vi "Untitled 10 (SubVI).vi"(6 "Fuel (kg/s)":dbl, 7 "PID gains":T1={"proportional gain (Kc)"=1.0, "integral time (Ti, min)"=0.01, "derivative time (Td, min)"=0.0} {"derivative time (Td, min)" format="%.3f"; "integral time (Ti, min)" format="%.3f"; "proportional gain (Kc)" format="%.3f"}, 9 "Fuel Control   (On/OFF)":bool, 10 "Numeric":dbl, 11 "Max T (K)":dbl) -> (3 "output":dbl)   [LabVIEW 2019]
uses:
  <vilib>/addons/control/pid/pid.llb/PID Advanced (DBL).vi
  <vilib>/addons/control/pid/NI_PID_pid.lvlib
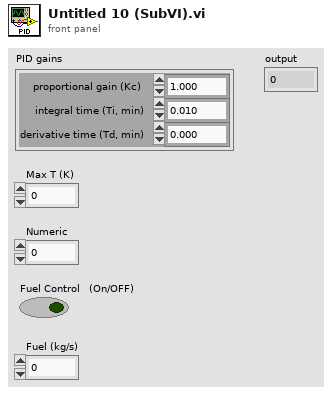
[diagram p1: front panel]
types:
  T1 = cluster{"proportional gain (Kc)":dbl, "integral time (Ti, min)":dbl, "derivative time (Td, min)":dbl}
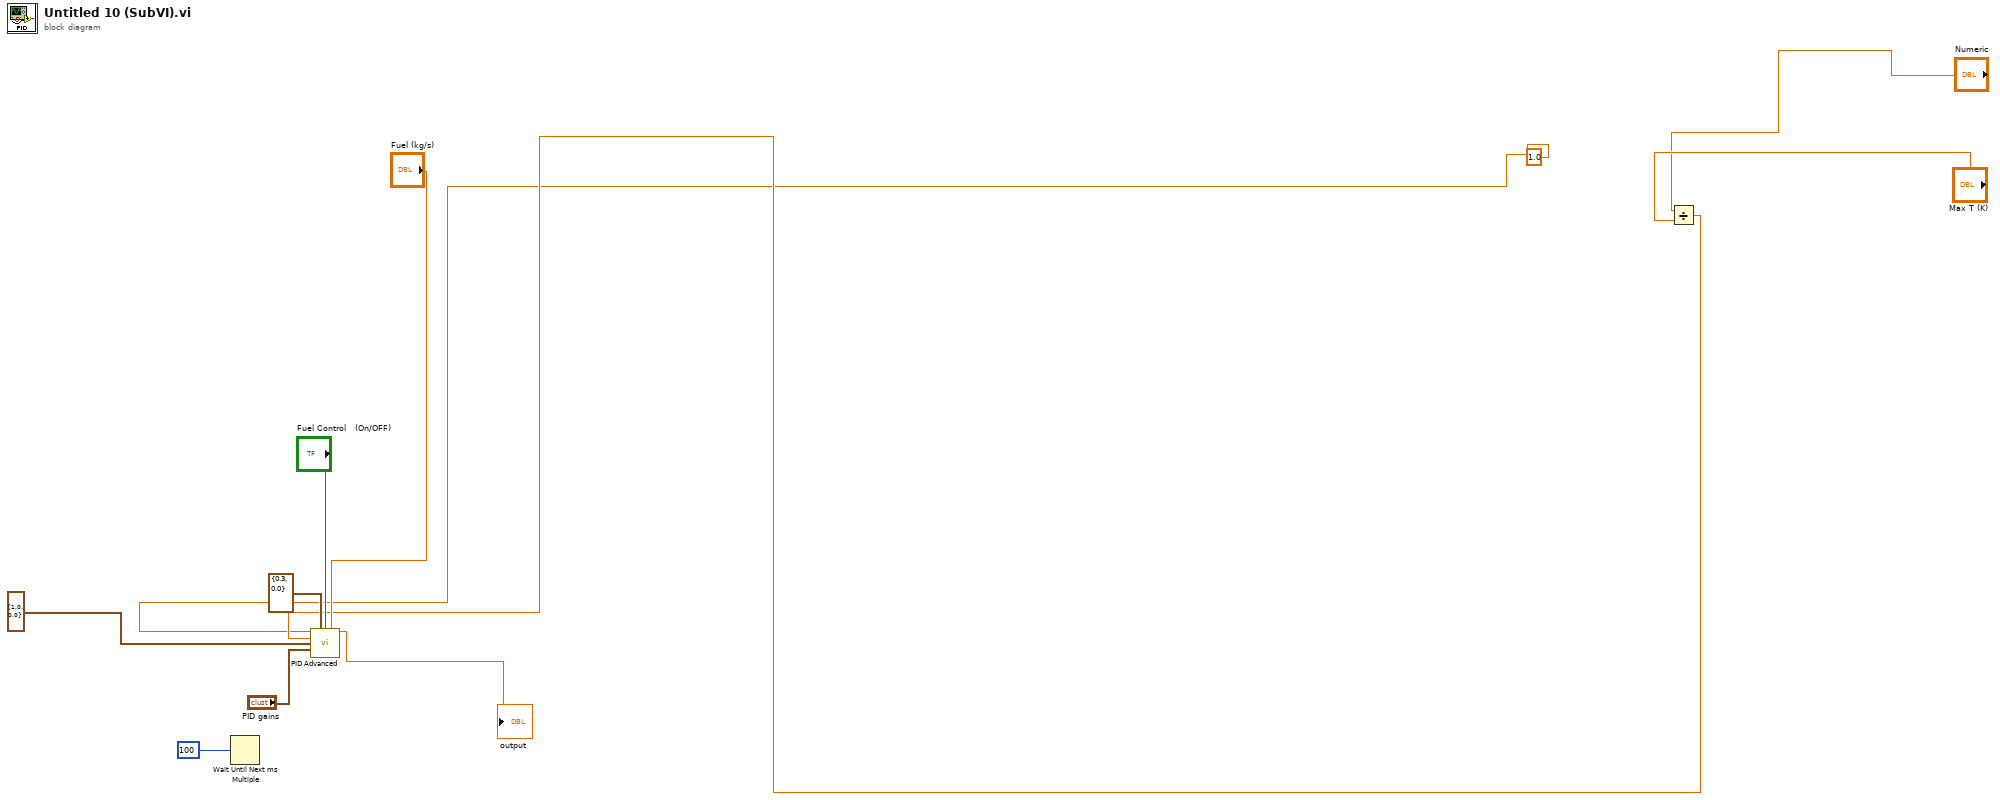
[diagram p0: block diagram]
diagram:
  n1 = Wait Until Next ms Multiple(millisecond multiple=100) -> ()  [unwired: 1 out]
  n2 = Divide(x="Numeric", y="Max T (K)") -> (x/y=w3:dbl)
  n3 = call-poly <vilib>:"PID Advanced.vi"("setpoint"=1.0, "output range"=cluster{"output high":dbl, "output low":dbl} {"output high"=0.3, "output low"=0.0}, "auto? (T)"="Fuel Control   (On/OFF)", "manual control"="Fuel (kg/s)", "process variable"=w3, "setpoint range"=cluster{"setpoint high":dbl, "setpoint low":dbl} {"setpoint high"=1.0, "setpoint low"=0.0}, "PID gains"="PID gains") -> ("output"=→"output":dbl)  [unwired: 7 in, 1 out]
